vi "Sensor_Values.vi"() -> ()   [LabVIEW 2019]
panel:
  in  "area_camera_target":dbl
  in  "y_camera_offset":dbl
  in  "x_camera_offset":dbl
  in  "Turret_Spin_Encoder":dbl
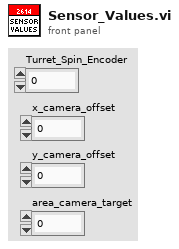
[diagram p1: front panel]
diagram:
